vi "Get Value.vi"(8 "error in (no error)":errorcluster, 11 "Refnum Value Source in":refnum<class "Path Ctrl Refnum.lvclass">) -> (0 "error out":errorcluster, 2 "Value":variant, 3 "Refnum Value Source out":refnum<class "Path Ctrl Refnum.lvclass">)   [LabVIEW 2020, in "Composed Columns.lvlib" / "Path Ctrl Refnum.lvclass"]
uses:
  Path Ctrl Refnum.lvclass
  Ctrl Renum Value Source Class/Ctrl Refnum Value Source.lvclass
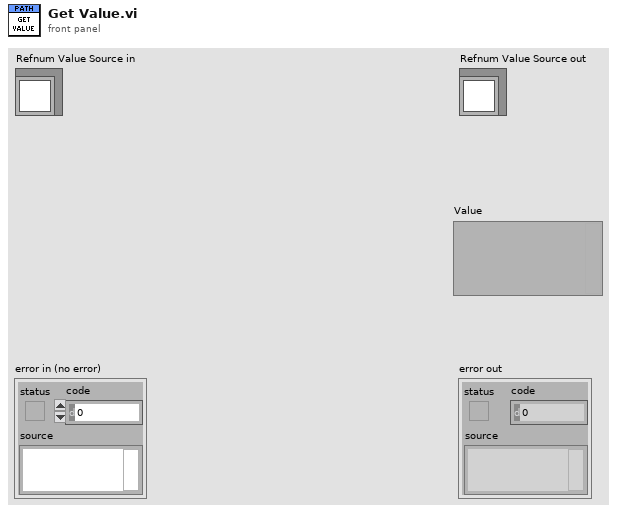
[diagram p1: front panel]
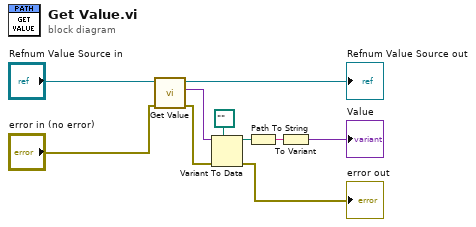
[diagram p0: block diagram]
diagram:
  n1 = call-parent "Get Value.vi"("error in (no error)"="error in (no error)", "Refnum Value Source in"="Refnum Value Source in") -> ("error out"=w3:errorcluster, "Value"=w8:variant, "Refnum Value Source out"=→"Refnum Value Source out":refnum<class "Path Ctrl Refnum.lvclass">)  [unwired: 7 in]
  n2 = Variant To Data(error in=w3, type=path "", Variant=w8) -> (data=w6:path, error out=→"error out":errorcluster)
  n3 = Path To String(path=w6) -> (string=w5:string)
  n4 = To Variant(anything=w5) -> (Variant=→"Value":variant)
